vi "Remove Key.vi"(7 "Section":string, 8 "error in (no error)":errorcluster, 10 "Key":string, 11 "Ini Path in":path) -> (0 "error out":errorcluster, 2 "Key Found?":bool, 3 "Ini Path out":path)   [LabVIEW 2021, in "Config.lvlib"]
uses:
  Config.lvlib
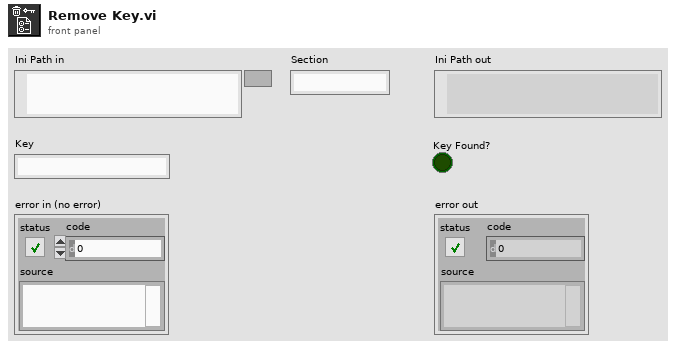
[diagram p1: front panel]
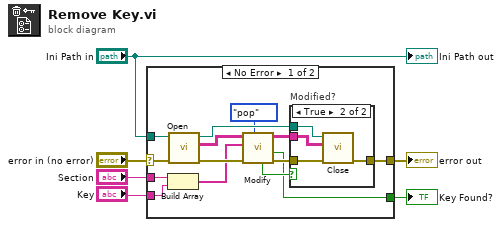
[diagram p0: block diagram]
diagram:
  n1 = case shown="No Error" "error in (no error)" {
    selector: "error in (no error)" -> [w18 w26]
    tunnel: "Section" -> [w20 _]
    tunnel: "Key" -> [w19 _]
    tunnel: [w15 w26] -> w3
    tunnel: [w8 _] -> w2
    tunnel: "Ini Path in" -> [w7 _]
    frame No Error {
      n2 = Build Array(w20, w19) -> (w10:string[])
      n3 = call "Open.vi"("error in (no error)"=w18, "Ini Path in"=w7) -> ("error out"=w17:errorcluster, "skvc out"=w14:string[][], "Ini Path out"=w13:path)  [unwired: 6 in, 1 out]
      n4 = call "Modify.vi"("Action (noop)"=enum8{"noop", "get", "set", "pop"}."pop", "error in (no error)"=w17, "skvc input"=w10, "skvc in"=w14) -> ("error out"=w16:errorcluster, "Found?"=w8:bool, "skvc out"=w12:string[][], "Modified?"=w9:bool)  [unwired: 3 in, 1 out]
      n5 = case "Modified?" shown="True" w9 {
        tunnel: w16 -> [w21 w25]
        tunnel: [w21 w24] -> w15
        tunnel: w13 -> [_ w23]
        tunnel: w12 -> [_ w22]
        frame False {
        }
        frame True {
          n6 = call "Close.vi"("error in (no error)"=w25, "skvc in"=w22, "Ini Path in"=w23) -> ("error out"=w24:errorcluster)  [unwired: 7 in, 1 out]
        }
      }
    }
    frame Error {
    }
  }
  "error out" <- w3
  "Key Found?" <- w2
  "Ini Path out" <- "Ini Path in"
